vi "testDevice.vi"(8 "error in (no error)":errorcluster, 11 "Device.lvclass":refnum<class "Device.lvclass">) -> (0 "error out":errorcluster)   [LabVIEW 2017, in "BridgePatternDemo.lvclass"]
uses:
  BridgePatternDemo.lvclass
  Device Class/Device.lvclass
  BasicRemote Class/BasicRemote.lvclass
  AdvancedRemote Class/AdvancedRemote.lvclass
  ConsoleOut/Print Options.ctl
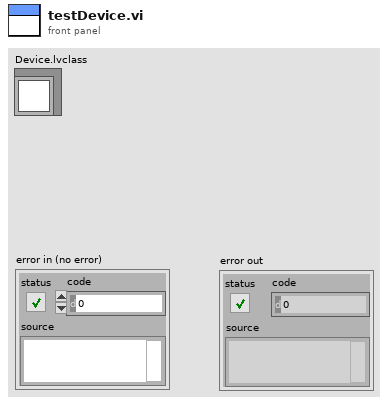
[diagram p1: front panel]
types:
  T1 = typedef "Print Options.ctl" = enum16{"Create", "Get Reference", "Print", "Print Header", "Close"}
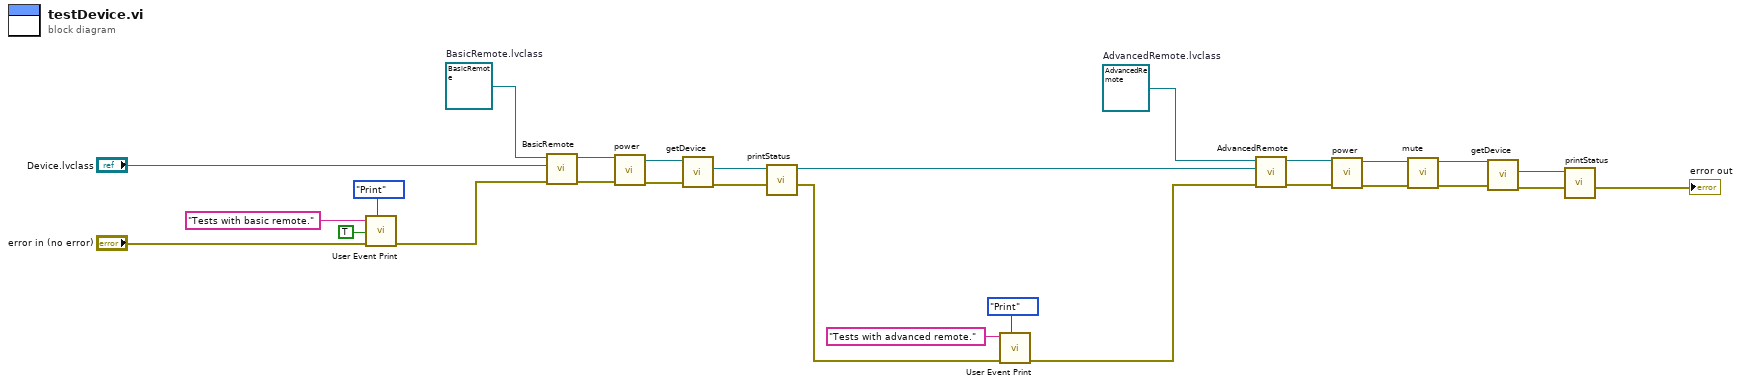
[diagram p0: block diagram]
diagram:
  w3 = refnum<class "AdvancedRemote.lvclass"> refnum  # AdvancedRemote.lvclass
  w14 = refnum<class "BasicRemote.lvclass"> refnum  # BasicRemote.lvclass
  n1 = call "User Event Print.vi"("Options"=Print_Options."Print", "error in (no error)"="error in (no error)", "add EOL? (T)"=TRUE ("add EOL?"), "String to Print"="Tests with basic remote." ("message")) -> ("error out"=w10:errorcluster)  [unwired: 6 in, 1 out]
  n2 = call-dynamic "BasicRemote.vi"("error in (no error)"=w10, "Device.lvclass"="Device.lvclass", "BasicRemote in"=w14) -> ("error out"=w27:errorcluster, "BasicRemote out"=w26:refnum<class "BasicRemote.lvclass">)  [unwired: 7 in]
  n3 = call-dynamic "power.vi"("error in (no error)"=w27, "BasicRemote in"=w26) -> ("error out"=w23:errorcluster, "BasicRemote out"=w24:refnum<class "BasicRemote.lvclass">)  [unwired: 8 in]
  n4 = call-dynamic "getDevice.vi"("error in (no error)"=w23, "BasicRemote in"=w24) -> ("error out"=w25:errorcluster, "Device.lvclass"=w2:refnum<class "Device.lvclass">)  [unwired: 7 in, 1 out]
  n5 = call-dynamic "printStatus.vi"("error in (no error)"=w25, "Device in"=w2) -> ("error out"=w6:errorcluster, "Device out"=w1:refnum<class "Device.lvclass">)  [unwired: 8 in]
  n6 = call "User Event Print.vi"("Options"=Print_Options."Print", "error in (no error)"=w6, "String to Print"="Tests with advanced remote." ("message")) -> ("error out"=w5:errorcluster)  [unwired: 7 in, 1 out]
  n7 = call-dynamic "AdvancedRemote.vi"("error in (no error)"=w5, "Device.lvclass"=w1, "AdvancedRemote in"=w3) -> ("error out"=w22:errorcluster, "AdvancedRemote out"=w21:refnum<class "AdvancedRemote.lvclass">)  [unwired: 7 in]
  n8 = call-dynamic "power.vi"("error in (no error)"=w22, "BasicRemote in"=w21) -> ("error out"=w18:errorcluster, "BasicRemote out"=w16:refnum<class "AdvancedRemote.lvclass">)  [unwired: 8 in]
  n9 = call-dynamic "mute.vi"("error in (no error)"=w18, "AdvancedRemote in"=w16) -> ("error out"=w17:errorcluster, "AdvancedRemote out"=w15:refnum<class "AdvancedRemote.lvclass">)  [unwired: 8 in]
  n10 = call-dynamic "getDevice.vi"("error in (no error)"=w17, "AdvancedRemote in"=w15) -> ("error out"=w20:errorcluster, "Device.lvclass"=w19:refnum<class "Device.lvclass">)  [unwired: 7 in, 1 out]
  n11 = call-dynamic "printStatus.vi"("error in (no error)"=w20, "Device in"=w19) -> ("error out"=→"error out":errorcluster)  [unwired: 8 in, 1 out]
